vi "主画面.vi"() -> ()   [LabVIEW 2016]
uses:
  <vilib>/Utility/sysdir.llb/System Directory Type.ctl
  <vilib>/Utility/config.llb/Read Key (String).vi
  <vilib>/Utility/config.llb/NI_LVConfig.lvlib
  data/FreeMem.dll
panel:
  in  "全屏":T1
  out "站点名称":string="站点名称"
  out "时间显示":string="2017-05-09 10:50:42"
  out "Version":string="Version:1.0.0"
  in  "主画面菜单":enum32{"首页", "数据查询", "运维调试", "系统设置"}(xcontrol)
  # "ESTD-XP 一体化水质自动监测系统"
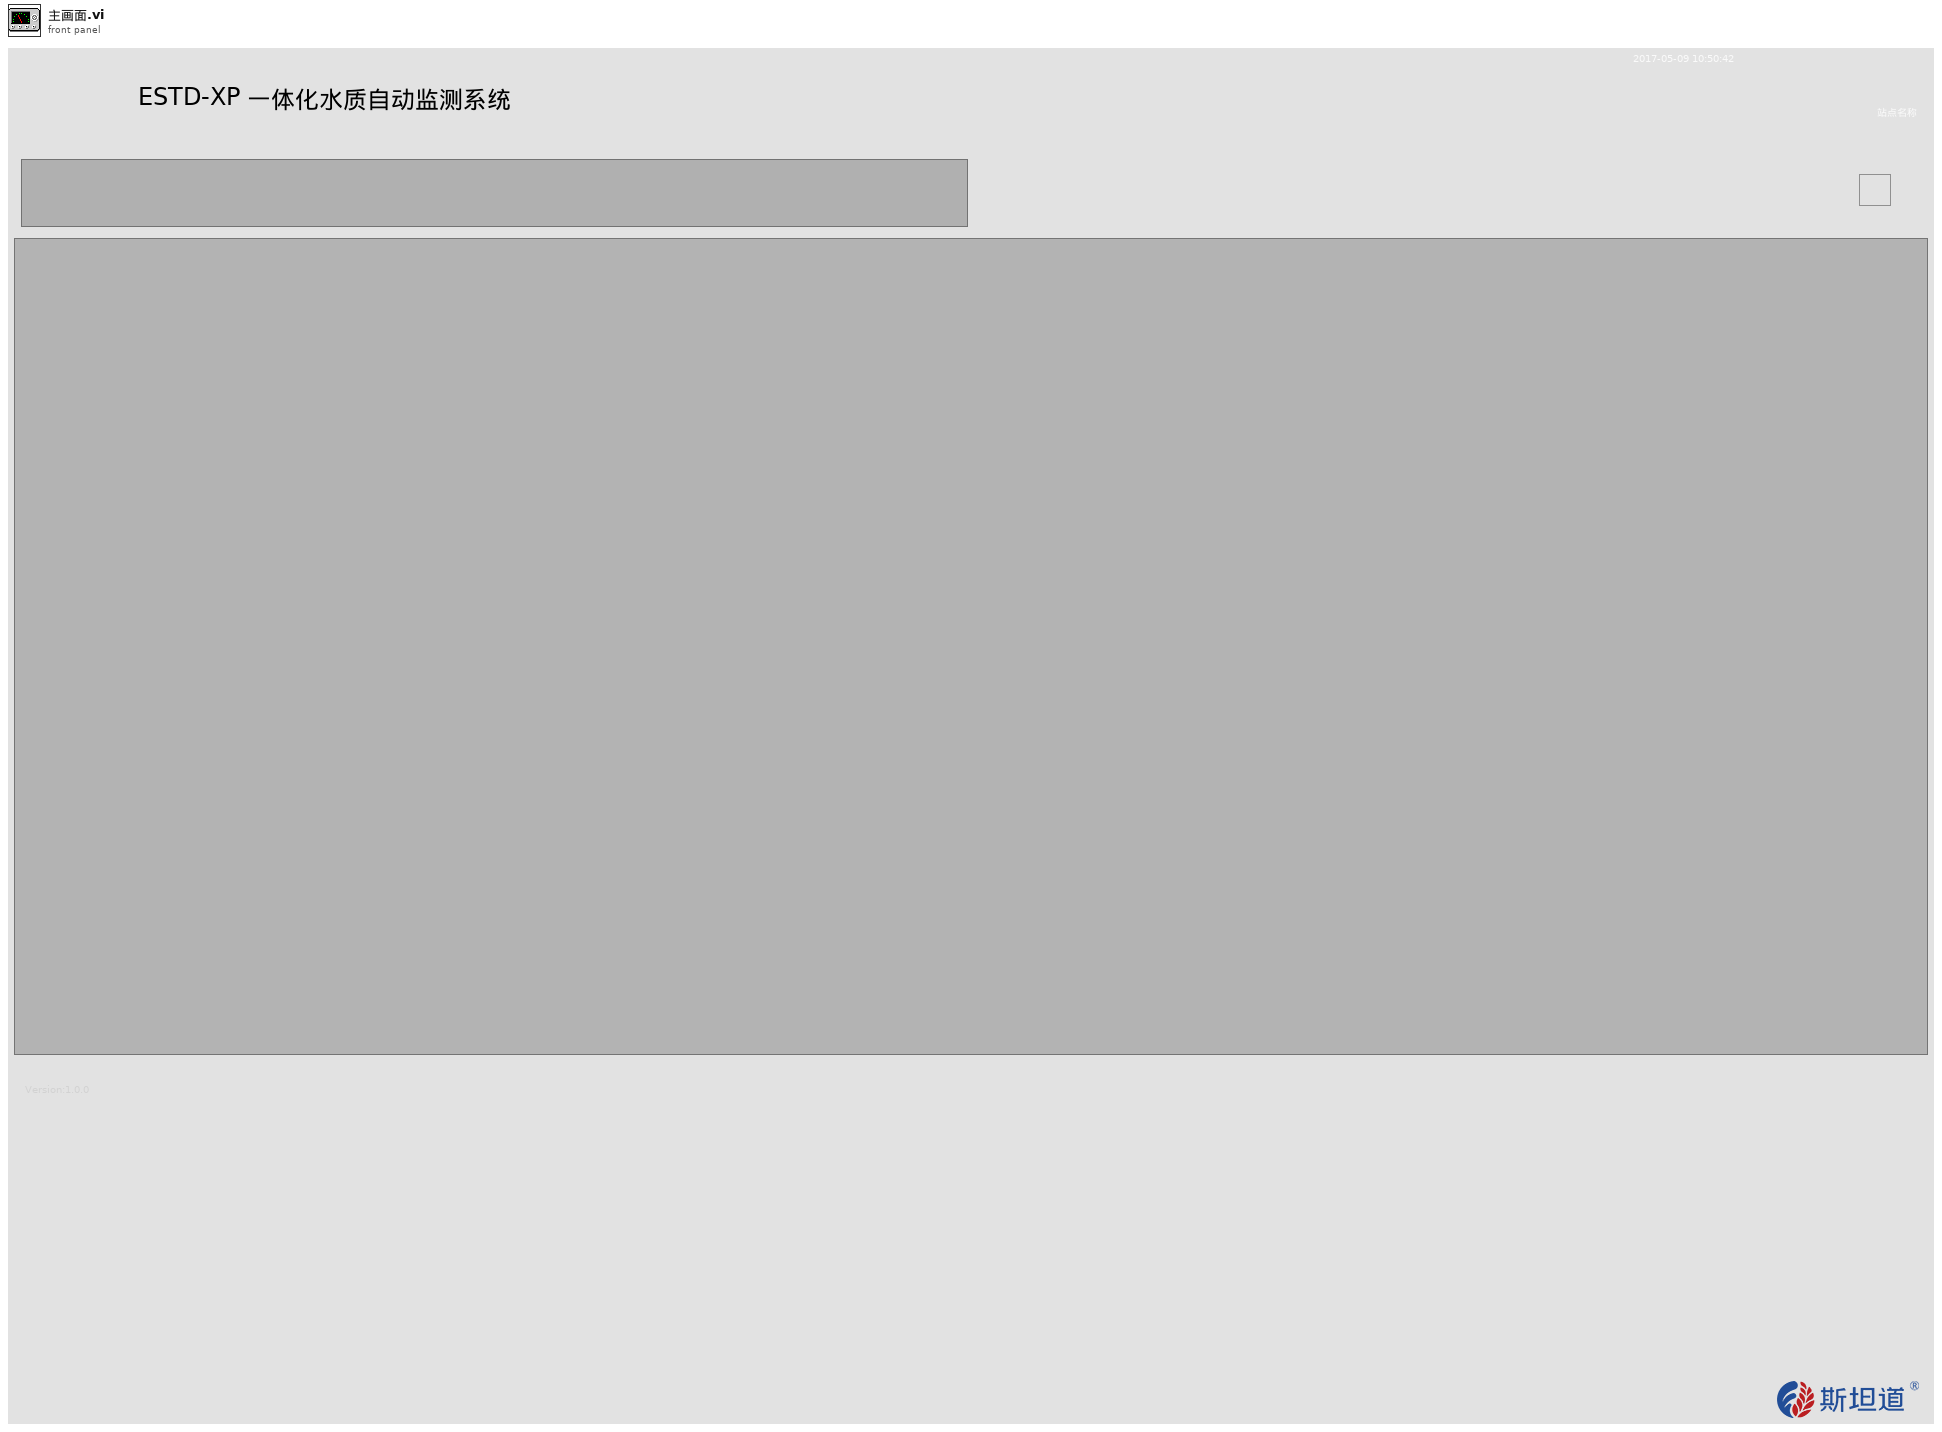
[diagram p1: front panel]
types:
  T1 = typedef "全屏按钮.ctl" = bool
  T2 = typedef "System Directory Type.ctl" = i32
  T3 = enum32{"Bad", "Idle", "Run top level", "Running"}
  T4 = cluster{"时间标识":timestamp, "设备":string, "日志信息":string, "流程参数":string}
  T5 = enum32{"invalid app kind", "Development System", "Run Time System", "Student Edition", "Embedded LabVIEW", "Evaluation", "Custom"}
  T6 = typedef "NI_LVConfig.lvlib/Config Data RefNum.ctl" = refnum<k1>
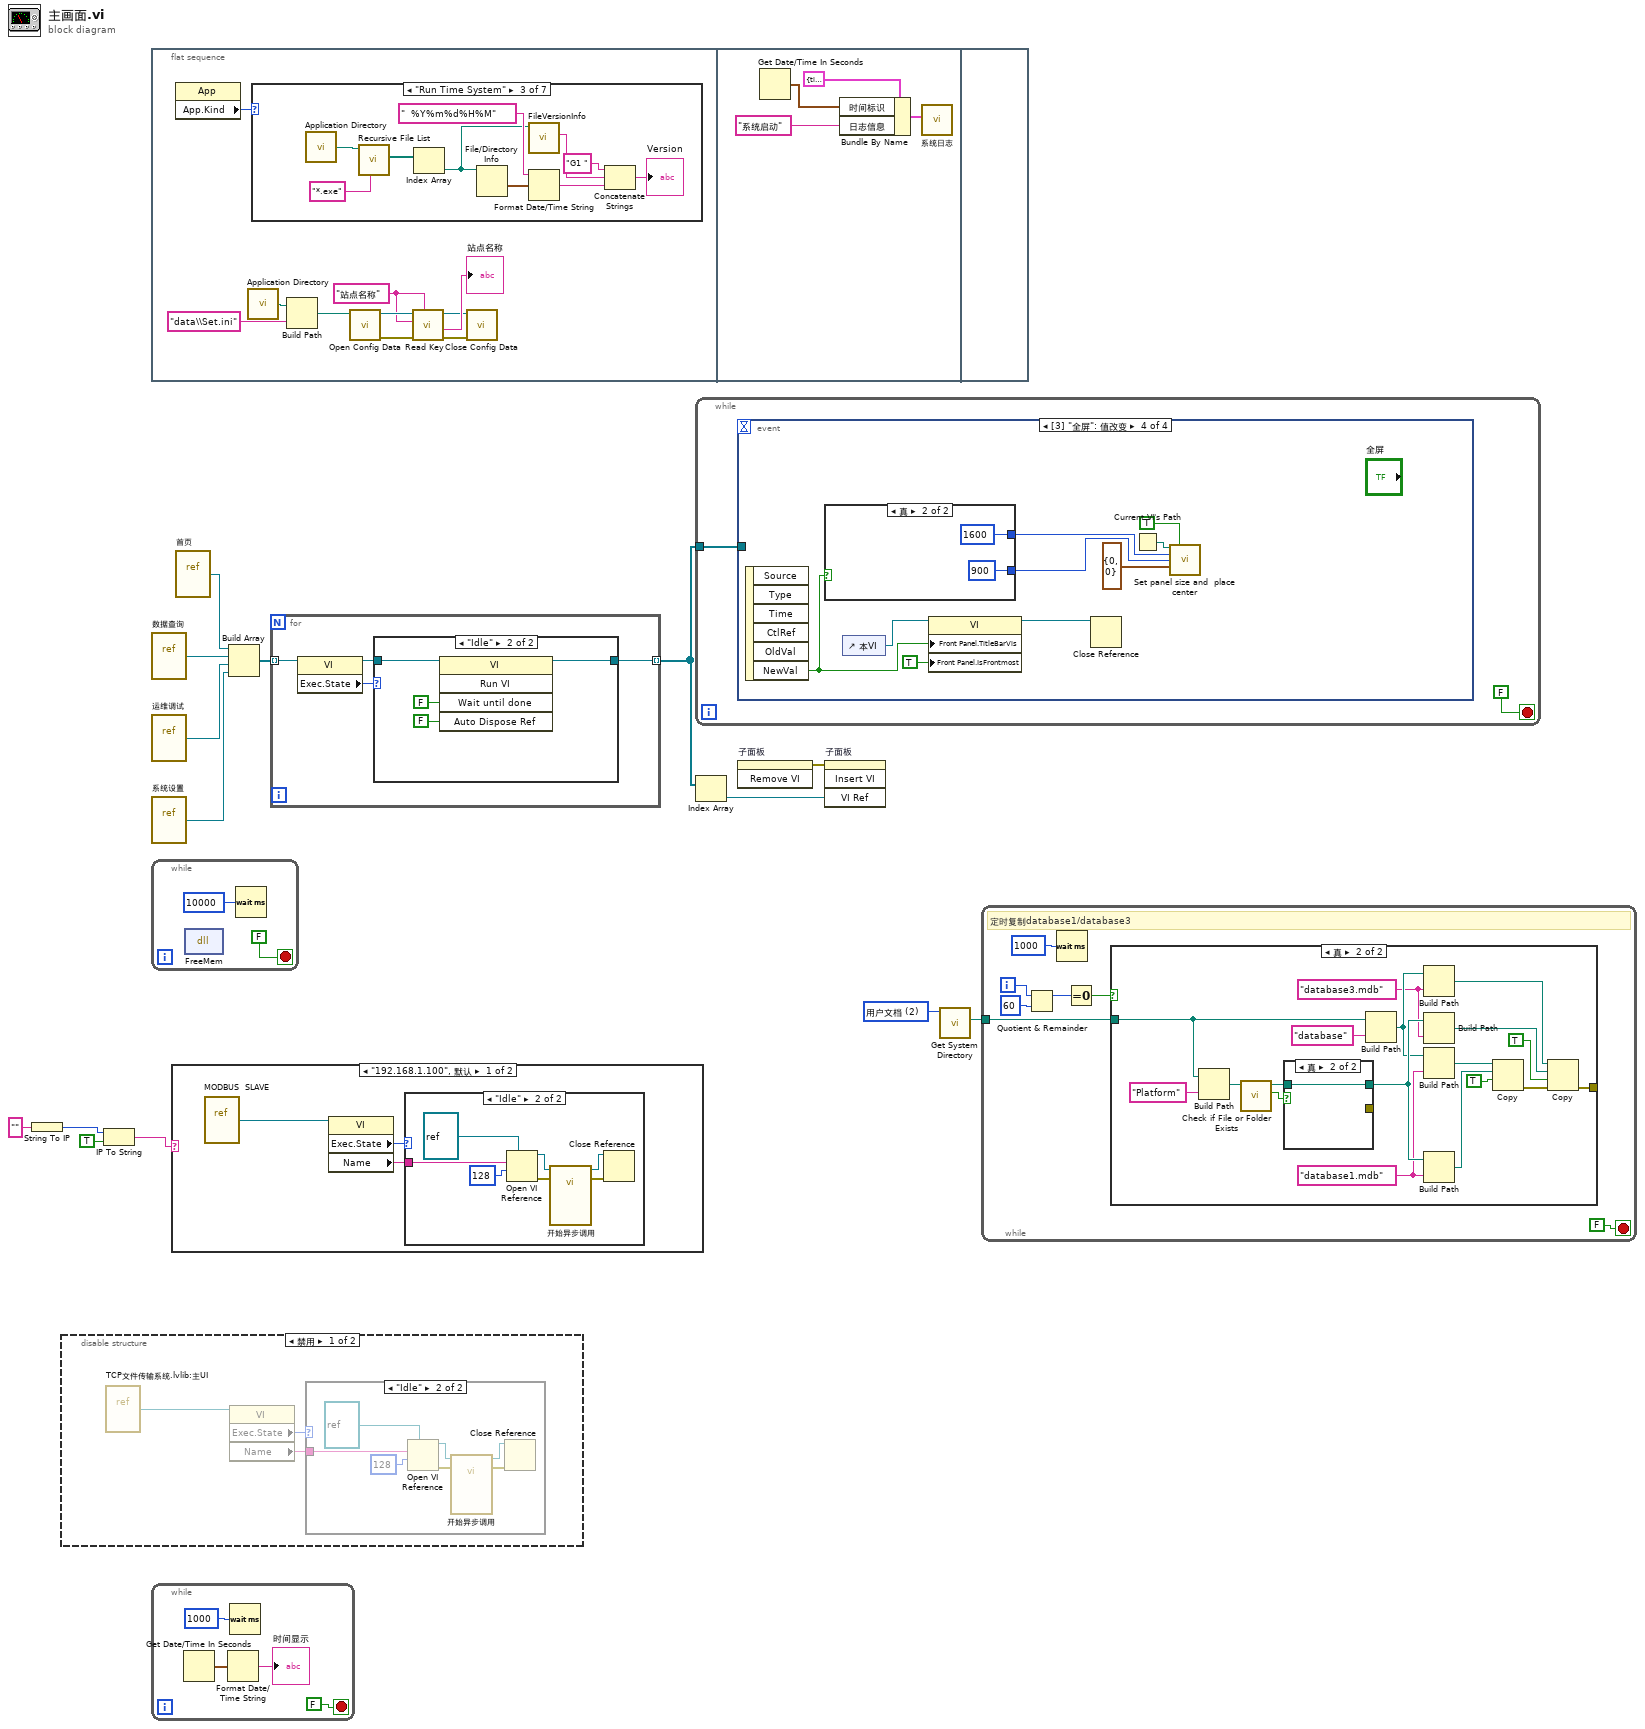
[diagram p0: block diagram]
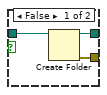
[diagram p7: hidden frame]
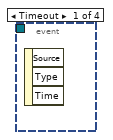
[diagram p15: hidden frame]
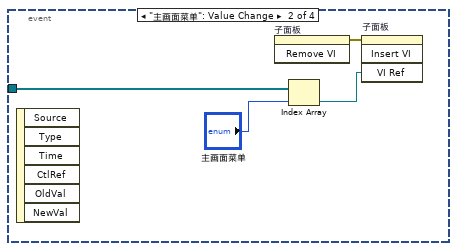
[diagram p16: hidden frame]
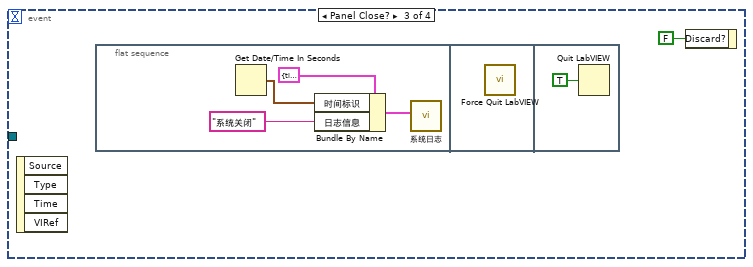
[diagram p17: hidden frame]
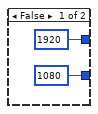
[diagram p18: hidden frame]
diagram:
  w6 = T2 2 items=["用户目录"=0, "用户桌面"=1, "用户文档"=2, "用户应用程序数据"=3, "用户设置"=4, "用户临时目录"=5, "公共文档"=6, "公共应用程序数据"=7, "公共设置"=8, "公共缓存"=13, "系统核心库"=9, "系统安装库"=10, "应用程序文件"=11, "启动盘根目录"=12] ("system directory type")
  n1 = String To IP(1:"" ("名称")) -> (0:w4:u32)
  n2 = disable-structure shown="禁用" {
    frame Disabled {
      n3 = vi-ref "TCP文件传输系统.lvlib:主UI.vi"() -> (w15:refnum<vi>)
      n4 = property class="VI"(reference=w15) -> ("Exec.State"=w16:T3, "Name"=w17:string)  [unwired: 1 in, 2 out]
      n5 = case shown="\"Idle\"" w16 {
        tunnel: w17 -> [_ w18]
        frame "Bad", Default {
        }
        frame "Idle" {
          n6 = Open VI Reference(type specifier VI Refnum (for type only)=refnum<vi> refnum, vi path=w18, options=128 ("选项")) -> (vi reference=w20:refnum<vi>, error out=w23:errorcluster)  [unwired: 3 in]
          n7 = call-by-ref "开始异步调用"(reference=w20, error in=w23) -> (reference out=w22:refnum<vi>, error out=w24:errorcluster)  [unwired: 12 in]
          n8 = Close Reference(reference=w22, error in (no error)=w24) -> ()  [unwired: 1 out]
        }
      }
    }
    frame Enabled {
    }
  }
  n9 = IP To String(1:TRUE ("句点符号？(F)"), 2:w4) -> (0:w1:string)
  n10 = flat-sequence {
    frame #0 {
      w25 = "站点名称" ("section")
      n11 = property class="App"() -> ("App.Kind"=w34:T5)  [unwired: 2 in, 2 out]
      n12 = call <vilib>:"Application Directory.vi"() -> ("Application Directory"=w28:path)
      n13 = case shown="\"Run Time System\"" w34 {
        frame "invalid app kind" {
        }
        frame "Development System", Default {
        }
        frame "Run Time System" {
          n14 = call <vilib>:"Application Directory.vi"() -> ("Application Directory"=w36:path)
          n15 = call <vilib>:"Recursive File List.vi"("pattern"="*.exe", "Folder Path"=w36) -> ("All Files in Dir"=w37:path[])  [unwired: 5 in, 4 out]
          n16 = Index Array(array=w37) -> (element=w35:path)  [unwired: 1 in]
          n17 = File/Directory Info(path=w35) -> (last mod=w41:timestamp)  [unwired: 1 in, 6 out]
          n18 = call <vilib>:"FileVersionInfo.vi"("Application Path in"=w35) -> ("File Version Info"=w43:string)  [unwired: 7 in, 3 out]
          n19 = Format Date/Time String(time format string (%c)="  %Y%m%d%H%M" ("时间格式字符串(%c)"), seconds (now)=w41) -> (date/time string=w39:string)  [unwired: 1 in]
          n20 = Concatenate Strings("G1 " ("字符串"), w43, w39) -> (→"Version":string)
        }
        frame "Student Edition" {
        }
        frame "Embedded LabVIEW" {
        }
        frame "Evaluation" {
        }
        frame "Custom" {
        }
      }
      n21 = Build Path(base path=w28, name or relative path="data\\Set.ini" ("名称或相对路径")) -> (appended path=w26:path)
      n22 = call <vilib>:"Open Config Data.vi"("configuration file path"=w26) -> ("error out"=w30:errorcluster, "refnum"=w33:T6)  [unwired: 8 in, 1 out]
      n23 = call-poly <vilib>:"Read Key.vi"("section"=w25, "error in (no error)"=w30, "key"=w25, "refnum"=w33) -> ("error out"=w29:errorcluster, "value"=→"站点名称":string, "refnum out"=w31:T6)  [unwired: 4 in, 1 out]
      n24 = call <vilib>:"Close Config Data.vi"("error in (no error)"=w29, "refnum"=w31) -> ()  [unwired: 8 in, 2 out]
    }
    frame #1 {
      n25 = Get Date/Time In Seconds() -> (seconds since 1Jan1904=w46:timestamp)
      n26 = Bundle By Name(cluster=T4 {"时间标识"=timestamp(0 s since 1904-01-01), "设备"="系统", "日志信息"="", "流程参数"=""} ("data in"), "时间标识"=w46, "日志信息"="系统启动") -> (w47:T4)
      n27 = call "系统日志.vi"("data in"=w47) -> ()  [unwired: 11 in]
    }
    frame #2 {
    }
  }
  n28 = vi-ref "数据查询.vi"() -> (w10:refnum<vi>)
  n29 = vi-ref "运维调试.vi"() -> (w9:refnum<vi>)
  n30 = vi-ref "系统设置.vi"() -> (w8:refnum<vi>)
  n31 = while {
    stop <- FALSE stop-if-true
    n32 = dll-call lib="PTH2mabs F\tgitkraken集成模板固定站（模板）!一体站项目 - 固定站模板dataFreeMem.dll" fn="FreeMem"() -> ()  [unwired: 4 in, 2 out]
    n33 = Wait (ms)(milliseconds to wait=u32 10000 ("等待时间（毫秒）")) -> ()  [unwired: 1 out]
  }
  n34 = while {
    stop <- FALSE stop-if-true
    n35 = Get Date/Time In Seconds() -> (seconds since 1Jan1904=w51:timestamp)
    n36 = Format Date/Time String(seconds (now)=w51) -> (date/time string=→"时间显示":string)  [unwired: 2 in]
    n37 = Wait (ms)(milliseconds to wait=u32 1000 ("等待时间（毫秒）")) -> ()  [unwired: 1 out]
  }
  n38 = case shown="\"192.168.1.100\", 默认" w1 {
    frame "192.168.1.100", Default {
      n39 = vi-ref "MODBUS  SLAVE.vi"() -> (w55:refnum<vi>)
      n40 = property class="VI"(reference=w55) -> ("Exec.State"=w56:T3, "Name"=w57:string)  [unwired: 1 in, 2 out]
      n41 = case shown="\"Idle\"" w56 {
        tunnel: w57 -> [_ w58]
        frame "Bad", Default {
        }
        frame "Idle" {
          n42 = Open VI Reference(type specifier VI Refnum (for type only)=refnum<vi> refnum, vi path=w58, options=128 ("选项")) -> (vi reference=w60:refnum<vi>, error out=w63:errorcluster)  [unwired: 3 in]
          n43 = call-by-ref "开始异步调用"(reference=w60, error in=w63) -> (reference out=w62:refnum<vi>, error out=w64:errorcluster)  [unwired: 11 in, 1 out]
          n44 = Close Reference(reference=w62, error in (no error)=w64) -> ()  [unwired: 1 out]
        }
      }
    }
    frame "192.168.1.101" {
    }
  }
  n45 = vi-ref "首页.vi"() -> (w11:refnum<vi>)
  n46 = Build Array(w11, w10, w9, w8) -> (w7:refnum<vi>[])
  n47 = for {
    tunnel: w7 -> [w68] mode=indexing
    tunnel: [w65] -> w13 mode=indexing
    n48 = property class="VI"(reference=w68) -> (reference out=w66:refnum<vi>, "Exec.State"=w67:T3)  [unwired: 1 in, 1 out]
    n49 = case shown="\"Idle\"" w67 {
      tunnel: w66 -> [w69 w71]
      tunnel: [w69 w70] -> w65
      frame "Bad", Default {
      }
      frame "Idle" {
        n50 = invoke class="VI" method="Run VI"(reference=w71, "Wait until done"=FALSE ("结束前等待"), "Auto Dispose Ref"=FALSE ("自动销毁引用")) -> (reference out=w70:refnum<vi>)  [unwired: 2 in, 4 out]
      }
    }
  }
  n51 = while {
    tunnel: w13 -> [w74]
    stop <- FALSE stop-if-true
    n52 = event shown="[3] \"全屏\": 值改变" {
      selector: _ -> [_ _ _ _]
      dyn-events: _ -> [_ _ _ _]
      timeout: _ -> [_ _ _ _]
      tunnel: w74 -> [_ w78 _ _]
      event Timeout {
        n53 = event-data() -> ()  [unwired: 1 in, 3 out]
      }
      event "主画面菜单": Value Change {
        n54 = event-data() -> ()  [unwired: 1 in, 6 out]
        n55 = invoke on="子面板" class="SubPnl" method="Remove VI"() -> (error out=w76:errorcluster)  [unwired: 3 in, 2 out]
        n56 = Index Array(array=w78, index="主画面菜单") -> (element=w77:refnum<vi>)
        n57 = invoke on="子面板" class="SubPnl" method="Insert VI"(error in=w76, "VI Ref"=w77) -> ()  [unwired: 2 in, 4 out]
      }
      event Panel Close? {
        n58 = event-data() -> ()  [unwired: 1 in, 4 out]
        n59 = flat-sequence {
          frame #0 {
            n60 = Get Date/Time In Seconds() -> (seconds since 1Jan1904=w83:timestamp)
            n61 = Bundle By Name(cluster=T4 {"时间标识"=timestamp(0 s since 1904-01-01), "设备"="系统", "日志信息"="", "流程参数"=""} ("data in"), "时间标识"=w83, "日志信息"="系统关闭") -> (w82:T4)
            n62 = call "系统日志.vi"("data in"=w82) -> ()  [unwired: 11 in]
          }
          frame #1 {
            n63 = call "Force Quit LabVIEW.vi"() -> ()  [unwired: 10 in, 2 out]
          }
          frame #2 {
            n64 = Quit LabVIEW(quit? (T)=TRUE ("退出？(T)")) -> ()
          }
        }
        n65 = event-data("Discard?"=FALSE ("放弃？")) -> ()  [unwired: 1 in, 1 out]
      }
      event Value Change {
        n66 = event-data() -> ("NewVal"=w89:T1)  [unwired: 1 in, 5 out]
        n67 = case shown="真" w89 {
          tunnel: [1920 ("Panel Width") 1600 ("Panel Width")] -> w88
          tunnel: [1080 ("Panel Height") 900 ("Panel Height")] -> w87
          frame False {
          }
          frame True {
          }
        }
        n68 = control-ref of="本VI"() -> (w94:refnum<vi>)
        n69 = property class="VI"(reference=w94, "Front Panel.TitleBarVis"=w89, "Front Panel.IsFrontmost"=TRUE ("前面板窗口:在最前")) -> (reference out=w90:refnum<vi>)  [unwired: 1 in, 1 out]
        n70 = Close Reference(reference=w90) -> ()  [unwired: 1 in, 1 out]
        n71 = Current VI's Path() -> (path=w93:path)
        n72 = call "Set panel size and  place center.vi"("Path"=w93, "Close Reference (false)"=TRUE, "Panel Width"=w88, "Panel Height"=w87, "FP.Origin in(H & V)"=cluster{"Horizontal":i16, "Vertical":i16} {"Horizontal"=0, "Vertical"=0}) -> ()  [unwired: 6 in, 5 out]
      }
    }
  }
  n73 = Index Array(array=w13) -> (element=w12:refnum<vi>)  [unwired: 1 in]
  n74 = invoke on="子面板" class="SubPnl" method="Remove VI"() -> (error out=w14:errorcluster)  [unwired: 3 in, 2 out]
  n75 = invoke on="子面板" class="SubPnl" method="Insert VI"(error in=w14, "VI Ref"=w12) -> ()  [unwired: 2 in, 4 out]
  n76 = call <vilib>:"Get System Directory.vi"("system directory type"=w6) -> ("system directory"=w5:path)  [unwired: 10 in]
  n77 = while {
    tunnel: w5 -> [w99]
    i -> [w103]
    stop <- FALSE stop-if-true
    # "定时复制database1/database3"
    n78 = Quotient & Remainder(x=w103, y=60) -> (x-y*floor(x/y)=w101:i32)  [unwired: 1 out]
    n79 = Wait (ms)(milliseconds to wait=u32 1000 ("等待时间（毫秒）")) -> ()  [unwired: 1 out]
    n80 = Equal To 0?(x=w101) -> (x = 0?=w100:bool)
    n81 = case shown="真" w100 {
      tunnel: w99 -> [_ w113]
      tunnel: [_ w109] -> _
      frame False {
      }
      frame True {
        w107 = "database1.mdb" ("名称或相对路径")
        w108 = "database3.mdb" ("名称或相对路径")
        n82 = Build Path(base path=w113, name or relative path="Platform" ("名称或相对路径")) -> (appended path=w120:path)
        n83 = call <vilib>:"Check if File or Folder Exists.vi"("path"=w120) -> ("file or folder exists?"=w119:bool, "dup path"=w118:path)  [unwired: 8 in, 1 out]
        n84 = case shown="真" w119 {
          tunnel: [w125 w127] -> w115
          tunnel: w118 -> [w126 w127]
          tunnel: [w124 _] -> _
          frame False {
            n85 = Create Folder(path (use dialog)=w126) -> (created path=w125:path, error out=w124:errorcluster)  [unwired: 2 in, 1 out]
          }
          frame True {
          }
        }
        n86 = Build Path(base path=w113, name or relative path="database" ("名称或相对路径")) -> (appended path=w111:path)
        n87 = Build Path(base path=w111, name or relative path=w108) -> (appended path=w110:path)
        n88 = Build Path(base path=w115, name or relative path=w108) -> (appended path=w114:path)
        n89 = Build Path(base path=w111, name or relative path=w107) -> (appended path=w112:path)
        n90 = Build Path(base path=w115, name or relative path=w107) -> (appended path=w117:path)
        n91 = Copy(9:TRUE ("覆盖(F)"), 10:w117, 11:w112) -> (0:w116:errorcluster)  [unwired: 2 in, 2 out]
        n92 = Copy(8:w116, 9:TRUE ("覆盖(F)"), 10:w114, 11:w110) -> (0:w109:errorcluster)  [unwired: 1 in, 2 out]
      }
    }
  }
